vi "Dispense on Baseplate.vi"() -> ()   [LabVIEW 2020]
uses:
  Classes/Workspace/Workspace.ctl
  Classes/Routine/Secure Syringe/SecureRelease Syringe.lvclass
  Classes/Workspace/Carrier Tray/Syringe Space/Syringe Space.lvclass
  Classes/Workspace/Carrier Tray/Assembly Tray.lvclass
  Classes/Routine/Dispense/CAD Dispense/8 Inch CAD Dispense.lvclass
  Classes/Routine/Secure Syringe/SecureRelease Syringe.lvclass/SecureRelease Syringe.ctl
  Classes/Routine/Secure Syringe/Write Type.vi
  Classes/Controller/Controller.lvclass
  Classes/Workspace/Fixture.lvclass
panel:
  out "Workspace":T1
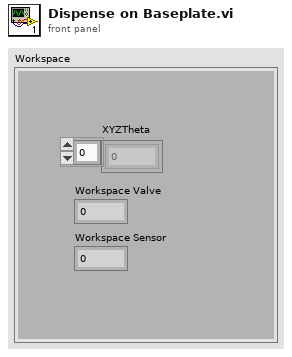
[diagram p1: front panel]
types:
  T1 = typedef "Fixture.lvclass/Workspace.ctl" = cluster{"XYZTheta":dbl[], "Workspace Valve":i32, "Workspace Sensor":i32}
  T2 = typedef "Controller.lvclass/Controllers.ctl" = cluster{"I-O.lvclass":refnum<class "I-O.lvclass">, "Dispenser.lvclass":refnum<class "Dispenser.lvclass">, "Gantry":refnum<k24>}
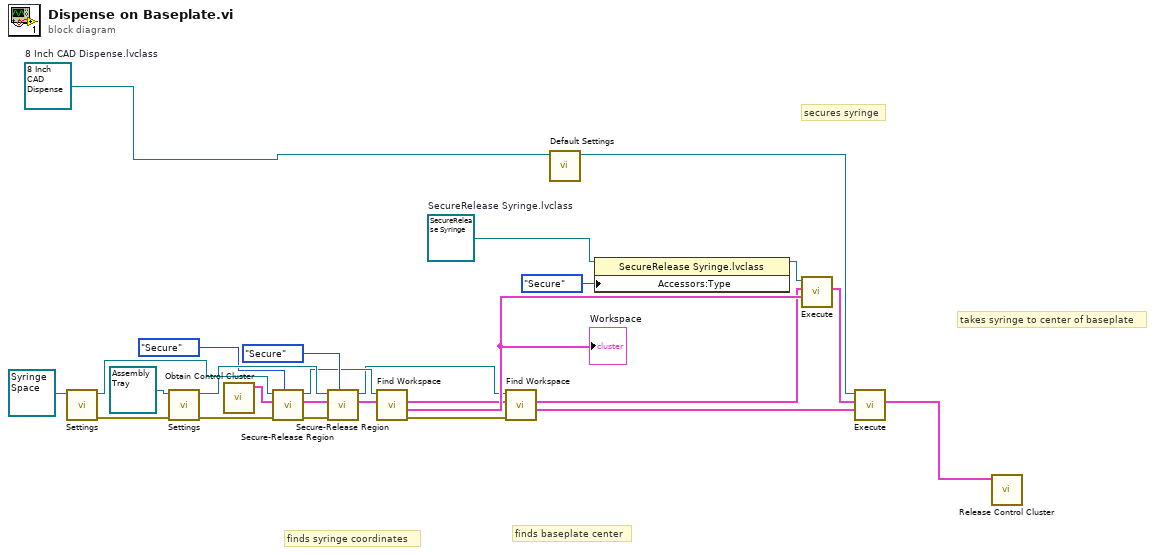
[diagram p0: block diagram]
diagram:
  w1 = refnum<class "8 Inch CAD Dispense.lvclass"> refnum  # 8 Inch CAD Dispense.lvclass
  w26 = refnum<class "SecureRelease Syringe.lvclass"> refnum  # SecureRelease Syringe.lvclass
  # "takes syringe to center of baseplate"
  # "finds baseplate center"
  # "secures syringe"
  # "finds syringe coordinates"
  n1 = call-dynamic "Settings.vi"("Syringe Space in"=refnum<class "Syringe Space.lvclass"> refnum ("Syringe Space.lvclass")) -> ("error out"=w11:errorcluster, "Syringe Space out"=w14:refnum<class "Syringe Space.lvclass">)  [unwired: 9 in]
  n2 = call-dynamic "Settings.vi"("error in (no error)"=w11, "Assembly Tray In"=refnum<class "Assembly Tray.lvclass"> refnum ("Assembly Tray.lvclass")) -> ("error out"=w10:errorcluster, "Assembly Tray Out"=w12:refnum<class "Assembly Tray.lvclass">)  [unwired: 8 in]
  n3 = call "Obtain Control Cluster.vi"() -> ("Control Out"=w6:T2)  [unwired: 11 in]
  n4 = call-dynamic "Secure-Release Region.vi"("Action"=enum16{"Secure", "Release"}."Secure", "error in (no error)"=w10, "Control In"=w6, "Carrier Tray in"=w14) -> ("error out"=w9:errorcluster, "Control Out"=w5:T2, "Carrier Tray out"=w3:refnum<class "Syringe Space.lvclass">)  [unwired: 5 in]
  n5 = call-dynamic "Secure-Release Region.vi"("Action"=enum16{"Secure", "Release"}."Secure", "error in (no error)"=w9, "Control In"=w5, "Carrier Tray in"=w12) -> ("Control Out"=w4:T2, "Carrier Tray out"=w2:refnum<class "Assembly Tray.lvclass">)  [unwired: 5 in, 1 out]
  n6 = call-dynamic "Find Workspace.vi"("Control In"=w4, "Carrier Tray in"=w3) -> ("Error Out"=w22:errorcluster, "Workspace"=w23:T1, "Control Out"=w19:T2)  [unwired: 6 in, 1 out]
  "Workspace" <- w23
  n7 = call-dynamic "Find Workspace.vi"("Error In"=w22, "Control In"=w19, "Carrier Tray in"=w2) -> ("Workspace"=w20:T1, "Control Out"=w18:T2)  [unwired: 5 in, 2 out]
  n8 = call-dynamic "Default Settings.vi"("8 Inch CAD Dispense in"=w1) -> ("8 Inch CAD Dispense out"=w16:refnum<class "8 Inch CAD Dispense.lvclass">)  [unwired: 9 in, 1 out]
  n9 = property class="SecureRelease Syringe.lvclass"(reference=w26, "Accessors:Type"=enum16{"Secure", "Remove"}."Secure" ("Type")) -> (reference out=w24:refnum<class "SecureRelease Syringe.lvclass">)  [unwired: 1 in, 1 out]
  n10 = call-dynamic "Execute.vi"("Workspace"=w23, "Control In"=w18, "Secure Syringe in"=w24) -> ("Control Out"=w21:T2)  [unwired: 6 in, 2 out]
  n11 = call-dynamic "Execute.vi"("Workspace"=w20, "Control In"=w21, "Dispense in"=w16) -> ("Control Out"=w17:T2)  [unwired: 6 in, 2 out]
  n12 = call "Release Control Cluster.vi"("output cluster"=w17) -> ()  [unwired: 11 in]
